vi "eliminateOutLierTriples.vi"(8 "error in (no error)":errorcluster, 10 "triplesWith\nSomeId":dbl[][](array[numeric]), 11 "Utilities in":refnum<class "Utilities.lvclass">) -> (0 "error out":errorcluster, 1 "std":T1, 2 "mean":T1, 3 "Utilities out":refnum<class "Utilities.lvclass">)   [LabVIEW 2021, in "Utilities.lvclass"]
uses:
  Utilities.lvclass
  Controls/RobotModel.ctl
  <vilib>/Analysis/NI_AALBase.lvlib
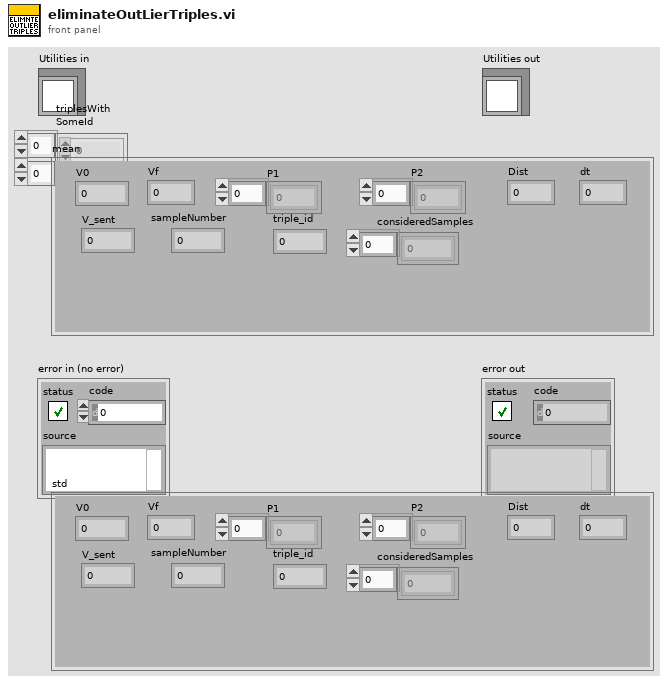
[diagram p1: front panel]
types:
  T1 = typedef "RobotModel.ctl" = cluster{"V0":dbl, "Vf":dbl, "Dist":dbl, "dt":dbl, "P1":dbl[], "P2":dbl[], "V_sent":dbl, "sampleNumber":i32, "triple_id":i32, "consideredSamples":dbl[]}
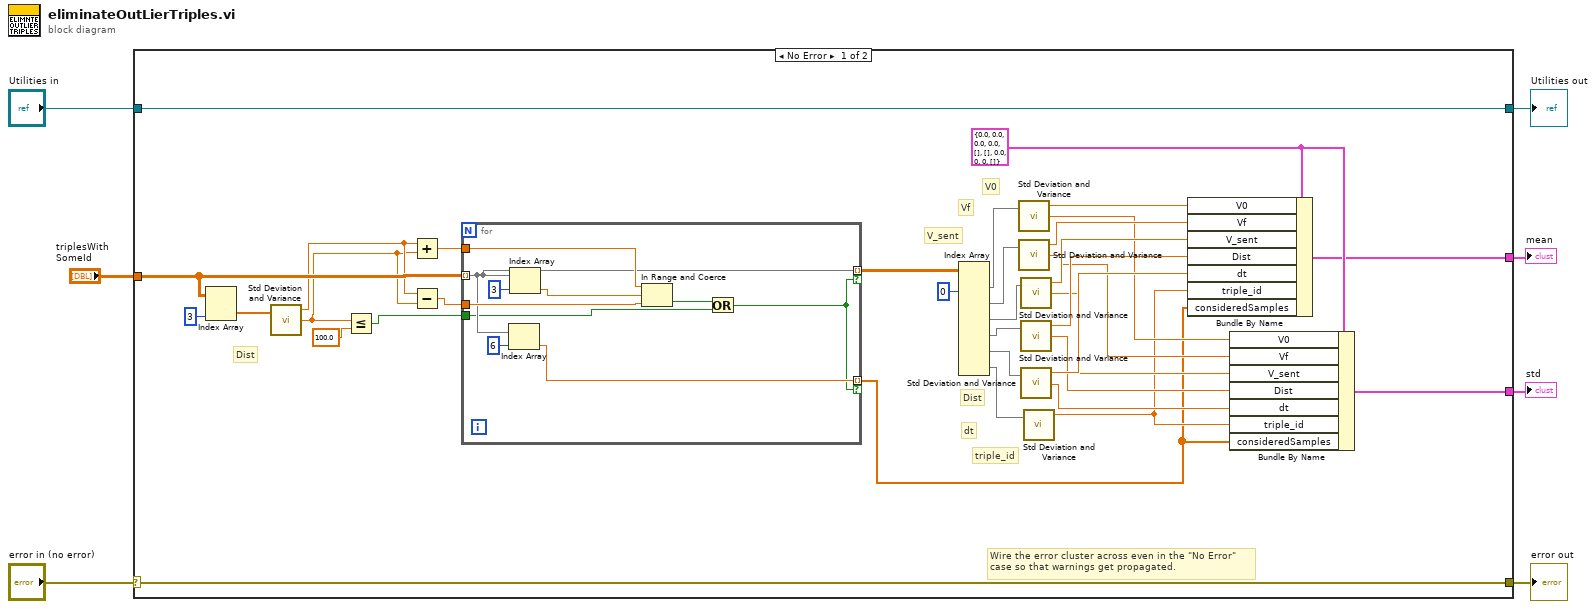
[diagram p0: block diagram]
diagram:
  n1 = case shown="No Error" "error in (no error)" {
    selector: "error in (no error)" -> [w40 w53]
    tunnel: [w40 w53] -> w6
    tunnel: [w41 w52] -> w4
    tunnel: "Utilities in" -> [w41 w52]
    tunnel: "triplesWith\nSomeId" -> [w17 _]
    tunnel: [w13 _] -> w2
    tunnel: [w12 _] -> w1
    frame No Error {
      w22 = T1 {"V0"=0.0, "Vf"=0.0, "Dist"=0.0, "dt"=0.0, "P1"=[], "P2"=[], "V_sent"=0.0, "sampleNumber"=0, "triple_id"=0, "consideredSamples"=[]} ("Robot Model")
      # "Dist"
      # "triple_id"
      # "dt"
      # "Dist"
      # "V_sent"
      # "Vf"
      # "V0"
      # "Wire the error cluster across even in the \"No Error\"\ncase so that warnings get propagated."
      n2 = Index Array(array=w17, index (col)=3 ("disabled index (col)")) -> (element=w19:dbl[])  [unwired: 1 in]
      n3 = call <vilib>:"Std Deviation and Variance.vi"("X"=w19) -> ("mean"=w16:dbl, "standard deviation"=w15:dbl)  [unwired: 1 in, 1 out]
      n4 = Less Or Equal?(x=w15, y=100.0) -> (x <= y?=w9:bool)
      n5 = Add(x=w16, y=w15) -> (x+y=w11:dbl)
      n6 = Subtract(x=w16, y=w15) -> (x-y=w10:dbl)
      n7 = for {
        tunnel: w17 -> [w47] mode=indexing
        tunnel: w11 -> [w49]
        tunnel: w10 -> [w48]
        tunnel: [w47] -> w14 mode=indexing if=w43
        tunnel: [w45] -> w8 mode=indexing if=w43
        tunnel: w9 -> [w42]
        n8 = Index Array(array=w47, index=6) -> (element=w45:dbl)
        n9 = Index Array(array=w47, index=3 ("disabled index (col)")) -> (element=w50:dbl)
        n10 = In Range and Coerce(upper limit=w49, x=w50, lower limit=w48) -> (In Range?=w44:bool)  [unwired: 1 out]
        n11 = Or(x=w44, y=w42) -> (x .or. y?=w43:bool)
      }
      n12 = Index Array(array=w14, index (col) #1=0 ("disabled index (col)")) -> (element #1=w38:dbl[], element #2=w37:dbl[], element #3=w36:dbl[], element #4=w35:dbl[], element #5=w34:dbl[], element #6=w33:dbl[])  [unwired: 11 in]
      n13 = call <vilib>:"Std Deviation and Variance.vi"("X"=w38) -> ("mean"=w32:dbl, "standard deviation"=w23:dbl)  [unwired: 1 in, 1 out]
      n14 = call <vilib>:"Std Deviation and Variance.vi"("X"=w37) -> ("mean"=w31:dbl, "standard deviation"=w24:dbl)  [unwired: 1 in, 1 out]
      n15 = call <vilib>:"Std Deviation and Variance.vi"("X"=w36) -> ("mean"=w30:dbl, "standard deviation"=w25:dbl)  [unwired: 1 in, 1 out]
      n16 = call <vilib>:"Std Deviation and Variance.vi"("X"=w35) -> ("mean"=w29:dbl, "standard deviation"=w26:dbl)  [unwired: 1 in, 1 out]
      n17 = call <vilib>:"Std Deviation and Variance.vi"("X"=w34) -> ("mean"=w28:dbl, "standard deviation"=w27:dbl)  [unwired: 1 in, 1 out]
      n18 = call <vilib>:"Std Deviation and Variance.vi"("X"=w33) -> ("mean"=w21:dbl)  [unwired: 1 in, 2 out]
      n19 = Bundle By Name(cluster=w22, "V0"=w32, "Vf"=w31, "V_sent"=w30, "Dist"=w29, "dt"=w28, "triple_id"=w21, "consideredSamples"=w8) -> (w13:T1)
      n20 = Bundle By Name(cluster=w22, "V0"=w23, "Vf"=w24, "V_sent"=w25, "Dist"=w26, "dt"=w27, "triple_id"=w21, "consideredSamples"=w8) -> (w12:T1)
    }
    frame Error {
    }
  }
  "error out" <- w6
  "Utilities out" <- w4
  "mean" <- w2
  "std" <- w1
